vi "Controllers.vi"(0 "FPGA Interface":refnum<k20>, 1 "error in (no error)":errorcluster, 2 "Yaw raw":dbl, 3 "Lean angle (deg) in":dbl, 4 "Path":dbl[](array[numeric]), 5 "Controller":enum32{"PID", "LQR"}(tab), 6 "Remote Control Data":T1, 7 "Reinitialize Balance PID":bool, 9 "K":dbl[](array[numeric]) format="%#_13g") -> (14 "FPGA VI Reference Out":refnum<k20>, 15 "error out":errorcluster, 16 "LQR direction":bool, 17 "Duty cycle (Only used for LQR)":dbl, 18 "Controller output":dbl, 19 "Signals to log":dbl[][](array[numeric]))   [LabVIEW 2016]
uses:
  Typedef/Remote Control Cluster.ctl
  <vilib>/Utility/error.llb/Error Cluster From Error Code.vi
  <vilib>/rvi/errors/niLvFpgaAdjustHostInterfaceError.vi
  <vilib>/addons/control/pid/pid.llb/PID (DBL).vi
  <vilib>/rvi/interface/nirviReadWriteControl/nirviReadWriteControl.xnode
  <vilib>/addons/control/pid/NI_PID_pid.lvlib
  NiFpgaLv.dll
  <vilib>/rvi/interface/Simulation/niFpgaSimulationCallBeginRW.vi
panel:
  # "8km/h PID gains\n\nP:   3.837\nI:   31.510\nD:  0.0022"
  # "LQR K-values\n\nK1:   37.3627\n\nK2:  -47.4259\nK3:    -8.6325\nK4:    15.8062"
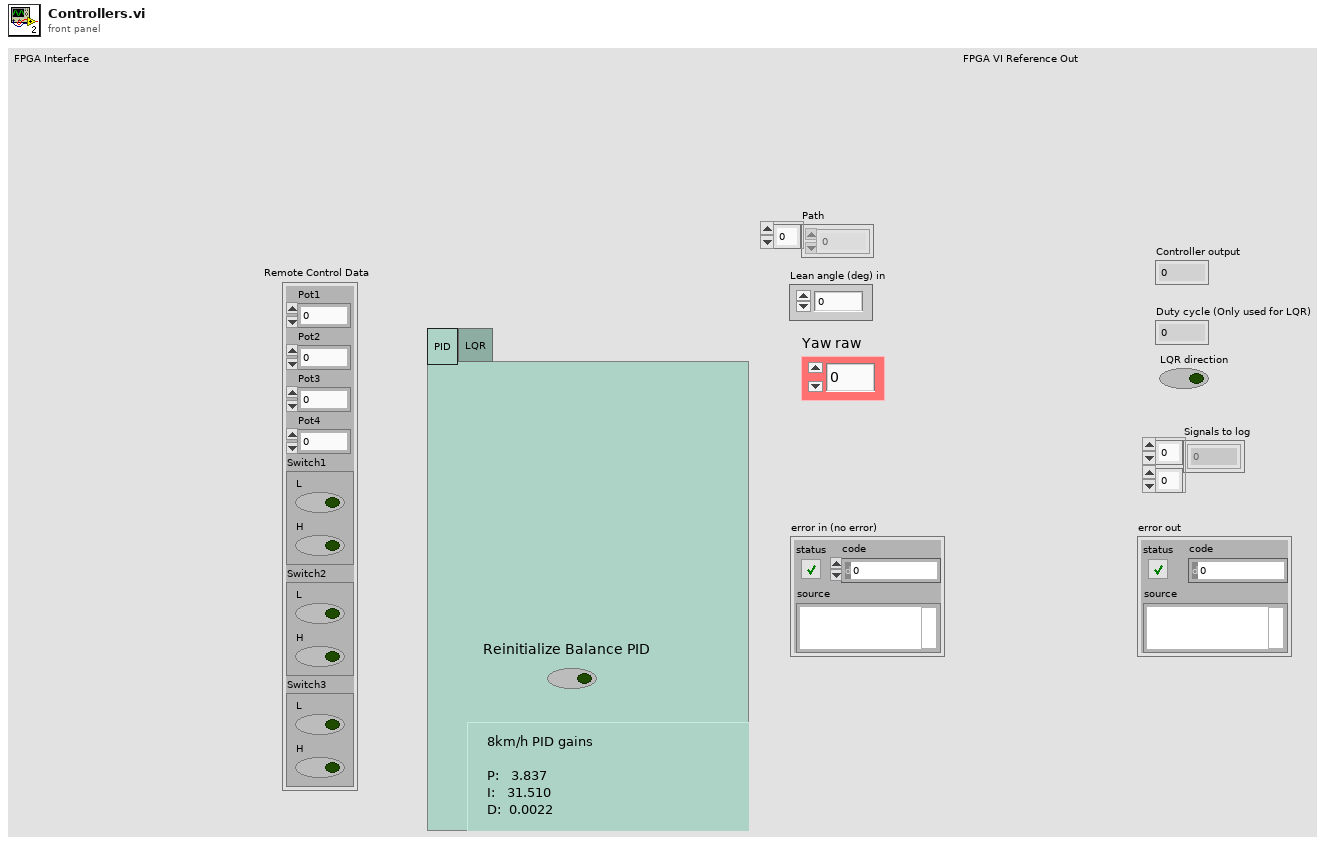
[diagram p1: front panel]
types:
  T1 = typedef "Remote Control Cluster.ctl" = cluster{"Pot1":u16, "Pot2":u16, "Pot3":u16, "Pot4":u16, "Switch1":cluster{"L":bool, "H":bool}, "Switch2":cluster{"L":bool, "H":bool}, "Switch3":cluster{"L":bool, "H":bool}}
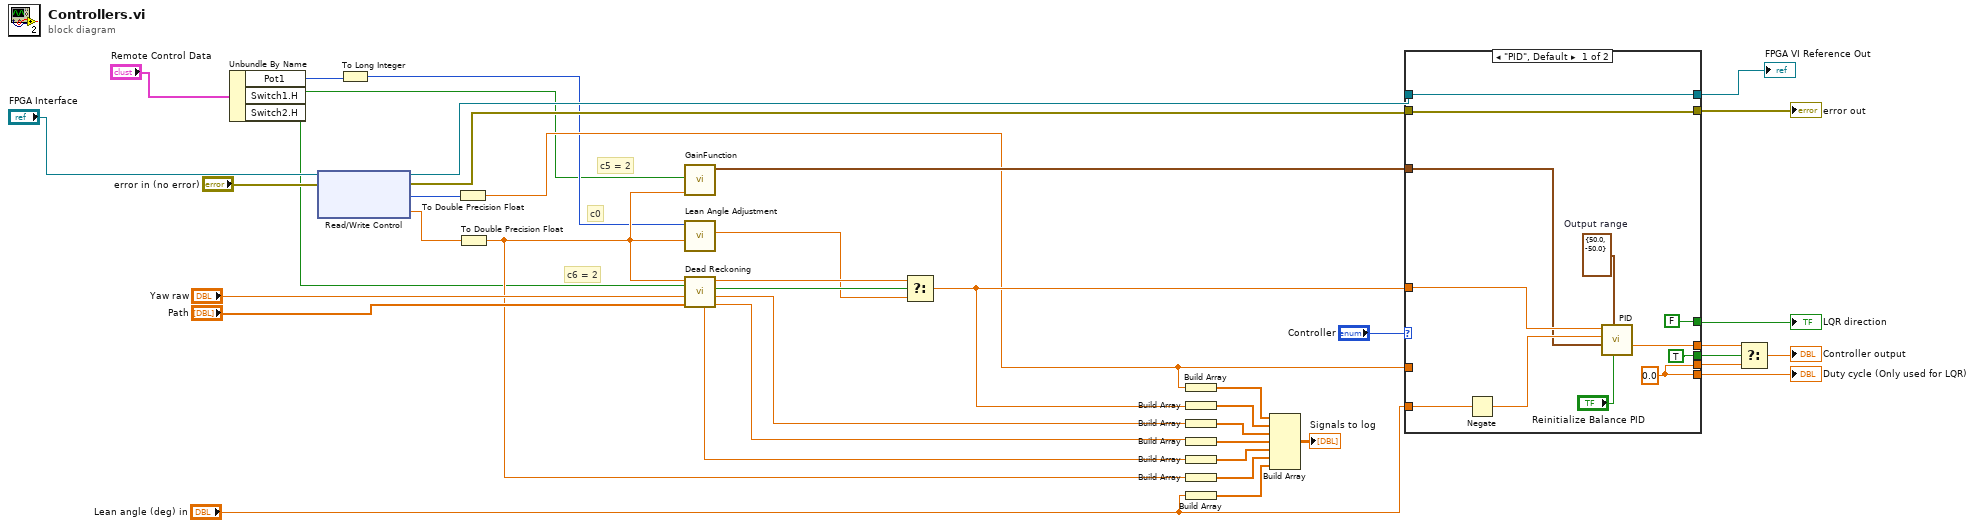
[diagram p0: block diagram]
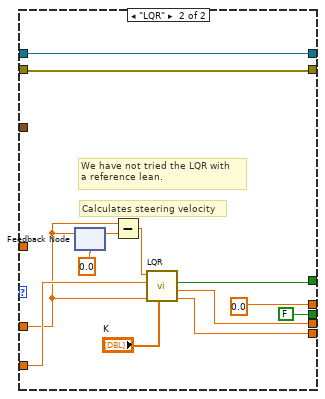
[diagram p2: hidden frame]
diagram:
  # "c5 = 2"
  # "c0"
  # "c6 = 2"
  n1 = Unbundle By Name("Remote Control Data") -> ("Pot1"=w5:u16, "Switch1.H"=w3:bool, "Switch2.H"=w2:bool)
  n2 = xnode "Read/Write Control"("FPGA VI Reference In"="FPGA Interface", "error in"="error in (no error)") -> ("FPGA VI Reference Out"=w25:refnum<k20>, "error out"=w38:errorcluster, "Position Axis1"=w1:i16, "Current speed"=w32:sgl)
  n3 = To Long Integer(number=w5) -> (32bit integer=w4:i32)
  n4 = To Double Precision Float(number=w1) -> (double precision float=w9:dbl)
  n5 = To Double Precision Float(number=w32) -> (double precision float=w20:dbl)
  n6 = call "GainFunction.vi"("Velocity"=w20, "Interpolate"=w3) -> ("PID gains"=w10:cluster{"P":dbl, "I":dbl, "D":dbl})  [unwired: 9 in]
  n7 = call "Lean Angle Adjustment.vi"("Velocity"=w20, "Value Channel 0"=w4) -> ("Reference lean angle"=w27:dbl)  [unwired: 9 in]
  n8 = call "Dead Reckoning.vi"("Path"="Path", "Yaw angle"="Yaw raw", "use PID"=w2, "Velocity"=w20) -> ("Yaw with offset"=w22:dbl, "Reference yaw"=w23:dbl, "Run dead reckoning?"=w29:bool, "Reference lean"=w28:dbl, "case"=w21:dbl)  [unwired: 3 in]
  n9 = Select(t=w28, s=w29, f=w27) -> (s? t:f=w24:dbl)
  n10 = Build Array(w9) -> (w17:dbl[])
  n11 = Build Array(w24) -> (w15:dbl[])
  n12 = Build Array(w23) -> (w12:dbl[])
  n13 = Build Array(w22) -> (w18:dbl[])
  n14 = Build Array(w21) -> (w13:dbl[])
  n15 = Build Array(w20) -> (w14:dbl[])
  n16 = Build Array("Lean angle (deg) in") -> (w16:dbl[])
  n17 = Build Array(w17, w15, w12, w18, w13, w14, w16) -> (→"Signals to log":dbl[][])
  n18 = case shown="\"PID\", Default" "Controller" {
    tunnel: "Lean angle (deg) in" -> [w43 w64]
    tunnel: [w50 0.0] -> w36
    tunnel: [FALSE ("Direction") w65] -> w33
    tunnel: [w48 w60] -> w35
    tunnel: w9 -> [_ w55]
    tunnel: [TRUE FALSE] -> w34
    tunnel: [w48 w57] -> w37
    tunnel: w24 -> [w47 _]
    tunnel: w38 -> [w45 w56]
    tunnel: [w45 w56] -> w39
    tunnel: w25 -> [w44 w54]
    tunnel: [w44 w54] -> w7
    tunnel: w10 -> [w42 _]
    frame "PID", Default {
      w53 = cluster{"output high":dbl, "output low":dbl} {"output high"=50.0, "output low"=-50.0}  # Output range
      w48 = 0.0 ("Duty cycle")
      n19 = Negate(x=w43) -> (-x=w52:dbl)
      n20 = call-poly <vilib>:"PID.vi"("reinitialize? (F)"="Reinitialize Balance PID", "output range"=w53, "PID gains"=w42, "process variable"=w52, "setpoint"=w47) -> ("output"=w50:dbl)  [unwired: 5 in, 1 out]
    }
    frame "LQR" {
      # "We have not tried the LQR with\na reference lean."
      # "Calculates steering velocity"
      n21 = feedback #1(0.0) -> (w62:dbl)
      n22 = feedback-in #1(w55) -> ()
      n23 = Subtract(x=w55, y=w62) -> (x-y=w59:dbl)
      n24 = call "LQR.vi"("K"="K", "Steering angle in"=w55, "Lean angle in"=w64, "Steering rate"=w59) -> ("Duty cycle"=w60:dbl, "Cout"=w57:dbl, "Direction"=w65:bool)  [unwired: 5 in]
    }
  }
  "error out" <- w39
  "Duty cycle (Only used for LQR)" <- w35
  "LQR direction" <- w33
  "FPGA VI Reference Out" <- w7
  n25 = Select(t=w36, s=w34, f=w37) -> (s? t:f=→"Controller output":dbl)
